vi "_Write XML Data.vi"(6 "Data (1D-I32)":i32[](array[numeric]), 7 "PrevString":string) -> (1 "Header":string, 3 "XML String":string)   [LabVIEW 2015]
uses:
  _Server Global.vi
panel:
  # "Raw Data:\nExpt#, Run Time in mS, data array in counts"
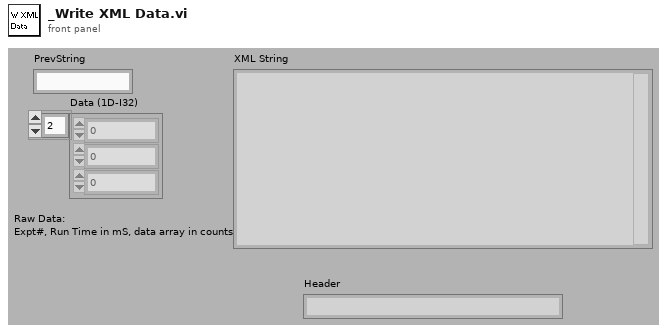
[diagram p1: front panel]
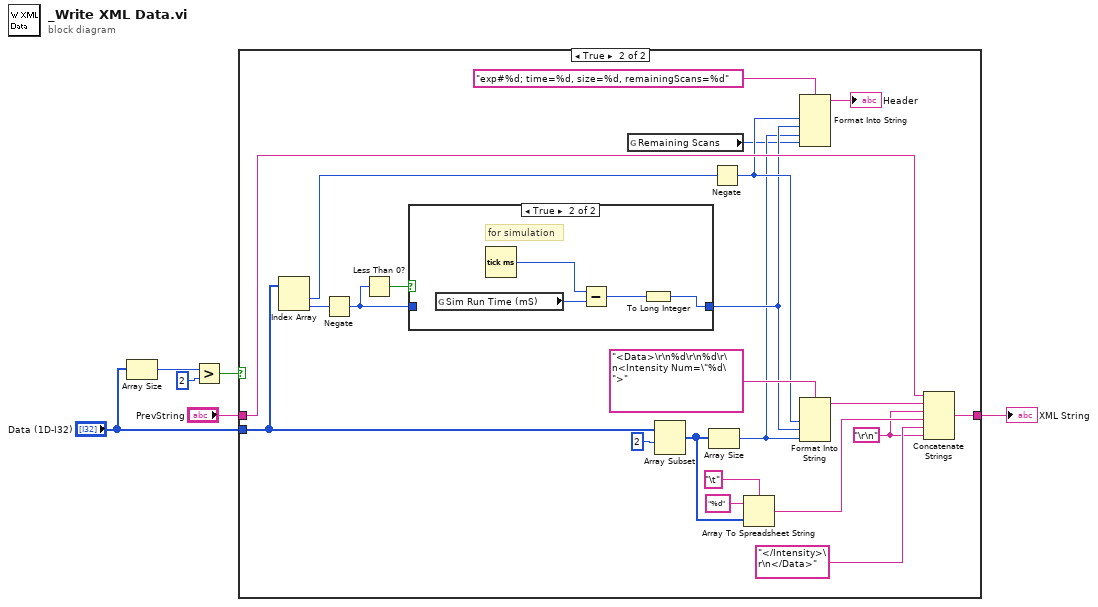
[diagram p0: block diagram]
diagram:
  n1 = Array Size(array="Data (1D-I32)") -> (size(s)=w4:i32)
  n2 = Greater?(x=w4, y=2) -> (0:w5:bool)
  n3 = case shown="True" w5 {
    tunnel: "Data (1D-I32)" -> [_ w21]
    tunnel: "PrevString" -> [w7 w14]
    tunnel: [w7 w13] -> w1
    frame False {
      # "No valid data received."
    }
    frame True {
      w19 = "\r\n"
      n4 = Index Array(array=w21) -> (element #1=w29:i32, element #2=w28:i32)  [unwired: 2 in]
      n5 = Negate(x=w28) -> (-x=w17:i32)
      n6 = Less Than 0?(x=w17) -> (x < 0?=w18:bool)
      n7 = case shown="True" w18 {
        tunnel: w17 -> [w30 _]
        tunnel: [w30 w33] -> w11
        frame False {
        }
        frame True {
          # "for simulation"
          n8 = global read "_Server Global.vi" "Sim Run Time (mS)"() -> (w31:u32)
          n9 = Tick Count (ms)() -> (millisecond timer value=w34:u32)
          n10 = Subtract(x=w34, y=w31) -> (x-y=w32:u32)
          n11 = To Long Integer(number=w32) -> (32bit integer=w33:i32)
        }
      }
      n12 = global read "_Server Global.vi" "Remaining Scans"() -> (w8:i32)
      n13 = Array Subset(array=w21, index=2) -> (w9:i32[])  [unwired: 1 in]
      n14 = Array Size(array=w9) -> (size(s)=w10:i32)
      n15 = Negate(x=w29) -> (-x=w12:i32)
      n16 = Array To Spreadsheet String(delimiter (Tab)="\t", array=w9, 3:"%d" ("format string")) -> (spreadsheet string=w22:string)
      n17 = Format Into String(format string="exp#%d; time=%d, size=%d, remainingScans=%d", w12, w11, w10, w8) -> (resulting string=→"Header":string)  [unwired: 2 in, 1 out]
      n18 = Format Into String(format string="<Data>\r\n%d\r\n%d\r\n<Intensity Num=\"%d\">", w12, w11, w10) -> (resulting string=w26:string)  [unwired: 2 in, 1 out]
      n19 = Concatenate Strings(w14, w26, w19, w22, "</Intensity>\r\n</Data>" ("format string"), w19) -> (w13:string)
    }
  }
  "XML String" <- w1
